vi "Test Process within App Log Error Message When Setting Handler After Process.vi"(8 "error in (no error)":errorcluster, 11 "Test Case In":refnum<class "Logger Test.lvclass">) -> (0 "error out":errorcluster, 3 "Test Case Out":refnum<class "Logger Test.lvclass">)   [LabVIEW 2020, in "Logger Test.lvclass"]
uses:
  Logger Test.lvclass
  C:/Program Files (x86)/National Instruments/LabVIEW 2020/vi.lib/Asteme/LUnit/Test Case.lvclass
  Mock Process/Mock Process.lvclass
  C:/Users/anton/Documents/GitHub/Triarc-Framework/source/Framework/Process/Process.lvclass
  C:/Users/anton/Documents/GitHub/Triarc-Framework/source/Framework/Logging/Logging.lvclass
  Framework/Application/Application.lvclass
  Mock Log Handler/Mock Log Handler.lvclass
  Framework/Process/Process.lvclass/Process.ctl
  Framework/Application/Application.lvclass/Application.ctl
  <vilib>/Asteme/LUnit/Test Case.lvclass/Test Case.ctl
  <vilib>/Asteme/LUnit/LUnit Assertion Result.lvclass/LUnit Assertion Result.ctl
  <vilib>/Asteme/LUnit/Palette/Pass.vi
  <vilib>/Asteme/LUnit/Palette/Fail.vi
  <vilib>/Asteme/LUnit/Variant to string.vi
  <vilib>/Asteme/LUnit/Set Assertion Type.vi
  Framework/Application/Private/Add Process to Map.vi
  Framework/Application/Private/Start Idle Processes if Running.vi
  Framework/Process/Protected/Messaging/Enqueue Message.vi
  Framework/Process/Public/Lifecycle/Get Lifecycle State.vi
  Framework/Process/Protected/SubVIs/Set Context.vi
  Framework/Process/Private/SubVIs/Wait for finish.vi
  Framework/Process/Private/SubVIs/Set Lifecycle State.vi
  Framework/Process/Protected/Messaging/Request Message.vi
  <vilib>/Asteme/LUnit/Add test result.vi
  <vilib>/Asteme/LUnit/LUnit Write Passed.vi
  <vilib>/Asteme/LUnit/LUnit Get Test Case.vi
  <vilib>/Asteme/LUnit/Assertion Result/LUnit Get Test Name.vi
  <vilib>/Asteme/LUnit/LUnit Write Message.vi
  <vilib>/Asteme/LUnit/LUnit Write Description.vi
  <vilib>/Asteme/LUnit/LUnit Write Assertion Type.vi
  Framework/Process/Public/Lifecycle/Leave Process Loop.vi
  Framework/Process/Private/SubVIs/Enqueue Request Message.vi
  <vilib>/Asteme/LUnit/Read Test Case Name.vi
  <vilib>/Utility/error.llb/Error Cluster From Error Code.vi
  Framework/Application/Private/Update Context for Owned Processes.vi
  Framework/Process/Private/SubVIs/Wait for Response Message.vi
  <vilib>/Utility/Data Type/Get Type Information.vi
  <vilib>/Utility/LVClass/Get LV Class Name.vi
  Framework/Process/Process.lvclass
  <vilib>/Asteme/LUnit/LUnit Assertion Result.lvclass
  Framework/Logging/Logging.lvclass
  <vilib>/Asteme/LUnit/Test Case.lvclass
  Support/Framework Test Support.lvlib
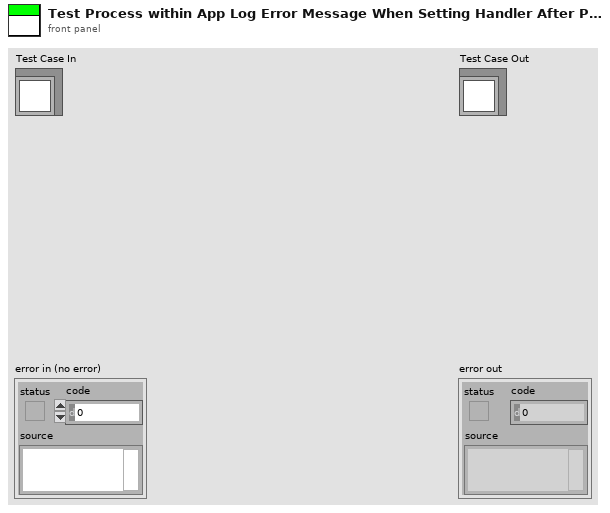
[diagram p1: front panel]
types:
  T1 = typedef "Mock Log Handler.lvclass/Log Entry.ctl" = cluster{"Level":string, "Source":string, "Message":string}
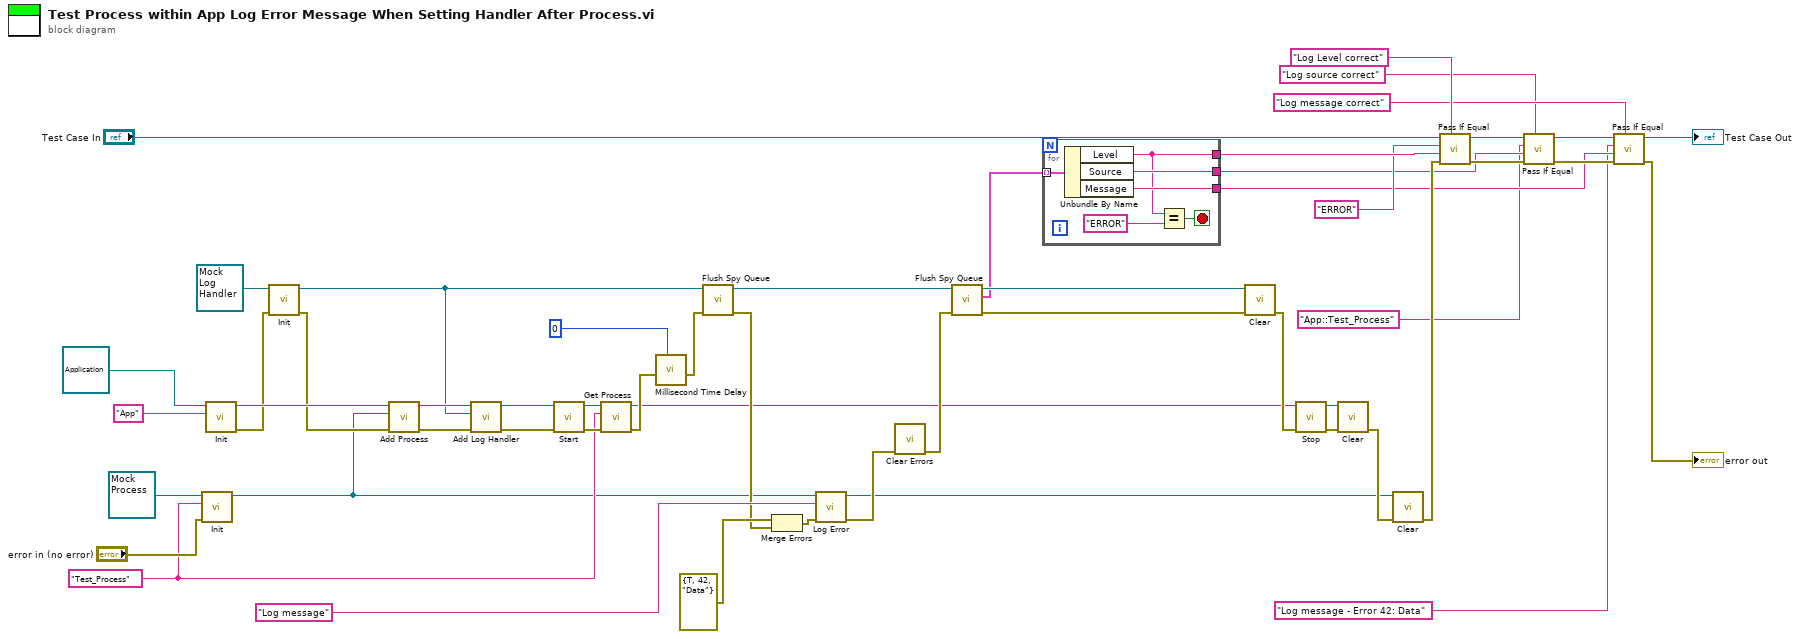
[diagram p0: block diagram]
diagram:
  w3 = "Test_Process" ("Name")
  n1 = call-dynamic "Init.vi"("error in (no error)"="error in (no error)", "Name"=w3, "Mock Process In"=refnum<class "Mock Process.lvclass"> refnum) -> ("Mock Process Out"=w2:refnum<class "Mock Process.lvclass">)  [unwired: 7 in, 1 out]
  n2 = call-dynamic "Init.vi"("Name"="App", "Process In"=refnum<class "Application.lvclass"> refnum ("Application.lvclass")) -> ("error out"=w47:errorcluster, "Process Out"=w50:refnum<class "Application.lvclass">)  [unwired: 8 in]
  n3 = call-dynamic "Init.vi"("error in (no error)"=w47, "Mock Log Handler In"=refnum<class "Mock Log Handler.lvclass"> refnum ("Mock Log Handler.lvclass")) -> ("error out"=w46:errorcluster, "Mock Log Handler Out"=w7:refnum<class "Mock Log Handler.lvclass">)  [unwired: 8 in]
  n4 = call "Add Process.vi"("error in (no error)"=w46, "Process"=w2, "Rig In"=w50) -> ("error out"=w20:errorcluster, "Rig Out"=w9:refnum<class "Application.lvclass">)  [unwired: 7 in]
  n5 = call "Add Log Handler.vi"("error in (no error)"=w20, "Log Handler"=w7, "Process In"=w9) -> ("error out"=w10:errorcluster, "Process Out"=w8:refnum<class "Application.lvclass">)  [unwired: 7 in]
  n6 = call "Start.vi"("error in (no error)"=w10, "Process In"=w8) -> ("error out"=w14:errorcluster, "Process Out"=w5:refnum<class "Application.lvclass">)  [unwired: 8 in]
  n7 = call "Get Process.vi"("error in (no error)"=w14, "Process Name"=w3, "Rig In"=w5) -> ("error out"=w6:errorcluster, "Rig Out"=w4:refnum<class "Application.lvclass">)  [unwired: 6 in, 1 out]
  n8 = call "Millisecond Time Delay.vi"("milliseconds to wait"=u32 0, "error in (no error)"=w6) -> ("error out"=w12:errorcluster)  [unwired: 7 in]
  n9 = call "Flush Spy Queue.vi"("error in (no error)"=w12, "Mock Log Handler in"=w7) -> ("error out"=w13:errorcluster, "Mock Log Handler out"=w15:refnum<class "Mock Log Handler.lvclass">)  [unwired: 7 in, 1 out]
  n10 = Merge Errors(errorcluster {"status"=TRUE, "code"=42, "source"="Data"} ("error in (no error)"), w13) -> (w17:errorcluster)
  n11 = call "Log Error.vi"("error in (no error)"=w17, "Message"="Log message", "Logging In"=w2) -> ("error out"=w27:errorcluster, "Logging Out"=w1:refnum<class "Mock Process.lvclass">)  [unwired: 7 in]
  n12 = call <vilib>:"Clear Errors.vi"("error in (no error)"=w27) -> ("error out"=w26:errorcluster)  [unwired: 5 in, 1 out]
  n13 = call "Flush Spy Queue.vi"("error in (no error)"=w26, "Mock Log Handler in"=w15) -> ("error out"=w44:errorcluster, "remaining elements"=w42:T1[], "Mock Log Handler out"=w45:refnum<class "Mock Log Handler.lvclass">)  [unwired: 7 in]
  n14 = for {
    tunnel: w42 -> [w59] mode=indexing
    tunnel: [w55] -> w41
    tunnel: [w58] -> w31
    tunnel: [w57] -> w30
    stop <- w54 stop-if-true
    n15 = Unbundle By Name(w59) -> ("Level"=w55:string, "Source"=w58:string, "Message"=w57:string)
    n16 = Equal?(x=w55, y="ERROR") -> (x = y?=w54:bool)
  }
  n17 = call-dynamic "Clear.vi"("error in (no error)"=w44, "Mock Log Handler In"=w45) -> ("error out"=w43:errorcluster)  [unwired: 9 in]
  n18 = call "Stop.vi"("error in (no error)"=w43, "Process In"=w4) -> ("error out"=w19:errorcluster, "Process Out"=w18:refnum<class "Application.lvclass">)  [unwired: 7 in, 1 out]
  n19 = call-dynamic "Clear.vi"("error in (no error)"=w19, "Application In"=w18) -> ("error out"=w49:errorcluster)  [unwired: 9 in]
  n20 = call-dynamic "Clear.vi"("error in (no error)"=w49, "Mock Process In"=w1) -> ("error out"=w35:errorcluster)  [unwired: 9 in]
  n21 = call <vilib>:"Pass If Equal.vi"("Description"="Log Level correct", "error in (no error)"=w35, "Actual"=w41, "Expected"="ERROR", "Test Case In"="Test Case In") -> ("error out"=w37:errorcluster, "Test Case Out"=w52:refnum<class "Logger Test.lvclass">)  [unwired: 5 in]
  n22 = call <vilib>:"Pass If Equal.vi"("Description"="Log source correct", "error in (no error)"=w37, "Actual"=w31, "Expected"="App::Test_Process" ("Name"), "Test Case In"=w52) -> ("error out"=w36:errorcluster, "Test Case Out"=w39:refnum<class "Logger Test.lvclass">)  [unwired: 5 in]
  n23 = call <vilib>:"Pass If Equal.vi"("Description"="Log message correct", "error in (no error)"=w36, "Actual"=w30, "Expected"="Log message - Error 42: Data" ("Message"), "Test Case In"=w39) -> ("error out"=→"error out":errorcluster, "Test Case Out"=→"Test Case Out":refnum<class "Logger Test.lvclass">)  [unwired: 5 in]
